vi "TestPulseGenerator.vi"() -> ()   [LabVIEW 2022 SP3, in "BinarySignalProcessClass.lvclass"]
uses:
  BinarySignalProcessClass.lvclass
panel:
  out "Waveform Chart":dbl[](graph)
  in  "TL":dbl
  in  "TH":dbl
  in  "stop":bool
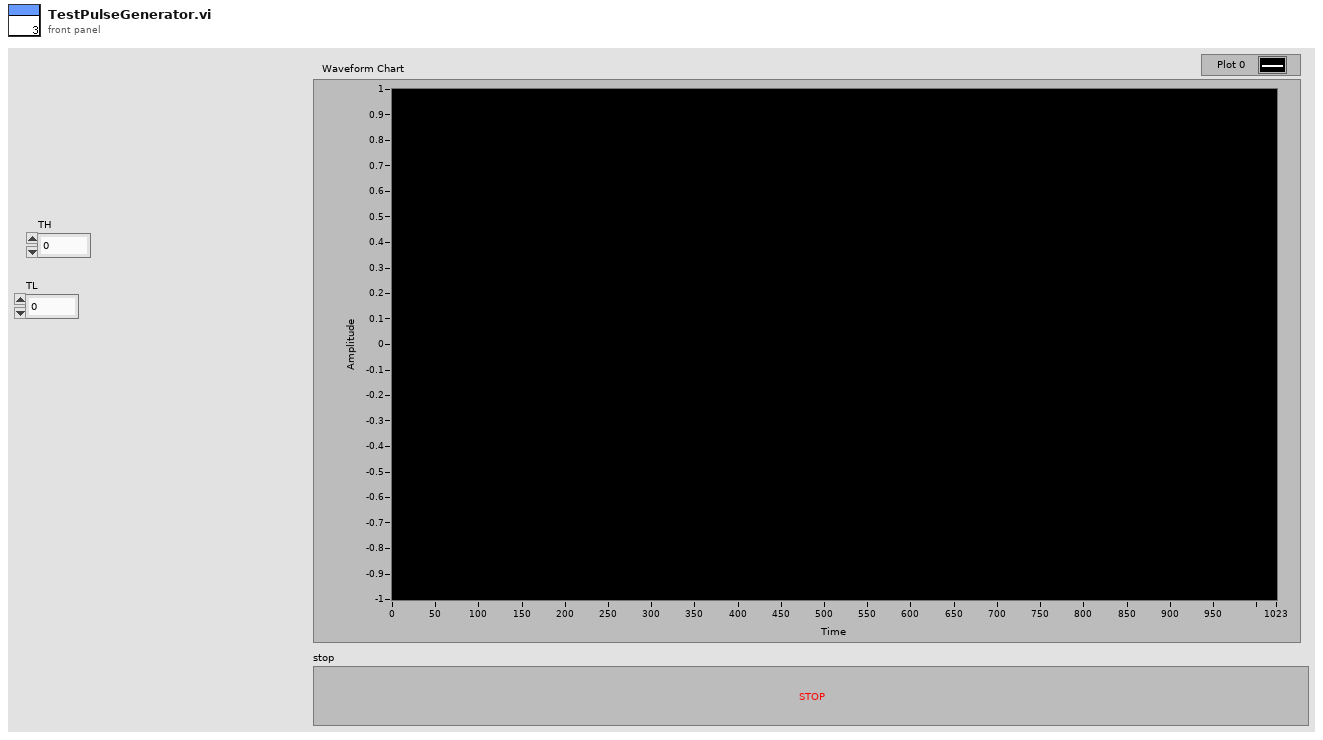
[diagram p1: front panel]
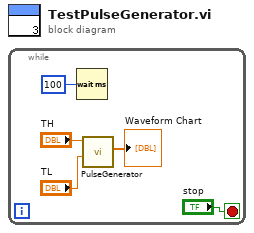
[diagram p0: block diagram]
diagram:
  n1 = while {
    stop <- "stop" stop-if-true
    n2 = Wait (ms)(milliseconds to wait=u32 100) -> ()  [unwired: 1 out]
    n3 = call "PulseGenerator.vi"("TL"="TL", "TH"="TH") -> ("Waveform Chart"=→"Waveform Chart":dbl[])  [unwired: 9 in]
  }
